vi "Verify.vi"(8 "error in (no error)":errorcluster, 10 "Comparator":refnum<class "Comparator.lvclass">, 11 "Mock In":refnum<class "Mock.lvclass">) -> (0 "error out":errorcluster, 1 "Errors":errorcluster[](array[cluster]), 2 "Results":cluster{"Passed?":bool, "Message":string}[](array[cluster]))   [LabVIEW 2020, in "Mock.lvclass"]
uses:
  Mock.lvclass
  Comparator/Comparator.lvclass
  Mock.lvclass/Mock.ctl
  Expectation/Expectation.lvclass
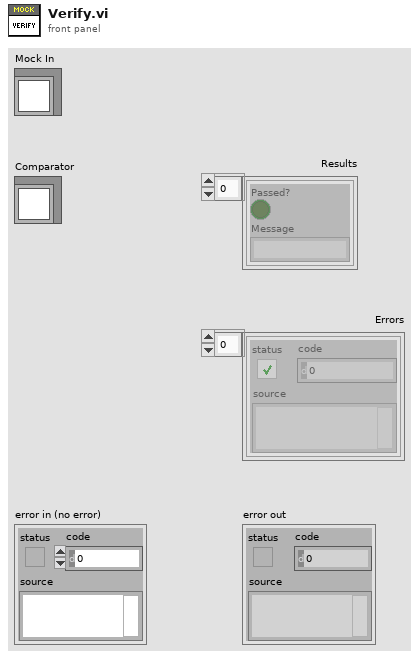
[diagram p1: front panel]
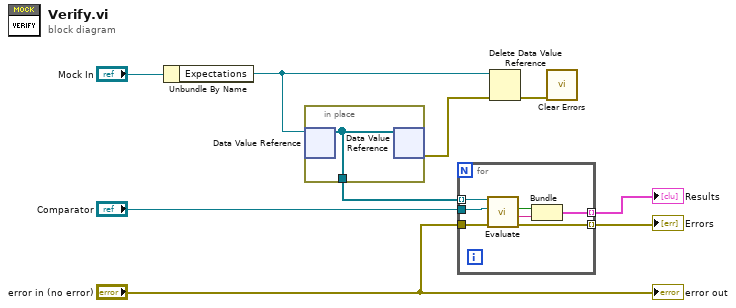
[diagram p0: block diagram]
diagram:
  n1 = Unbundle By Name("Mock In") -> ("Expectations"=w3:refnum<data-value>)
  n2 = in-place {
    in-place-border: [w10] -> w4
    n3 = in-place-dvr #1(w3) -> (w10:refnum<class "Expectation.lvclass">[])  [unwired: 1 out]
    n4 = in-place-dvr #1(w10) -> (w2:errorcluster)  [unwired: 1 out]
  }
  n5 = for {
    tunnel: "error in (no error)" -> [w17]
    tunnel: [w16] -> w7 mode=indexing
    tunnel: w4 -> [w15] mode=indexing
    tunnel: [w12] -> w6 mode=indexing
    tunnel: "Comparator" -> [w11]
    n6 = call-dynamic "Evaluate.vi"("error in (no error)"=w17, "Comparator"=w11, "Expectation in"=w15) -> ("error out"=w16:errorcluster, "Message"=w13:string, "Passed?"=w14:bool)  [unwired: 6 in]
    n7 = Bundle("Passed?"=w14, "Message"=w13) -> (w12:cluster{"Passed?":bool, "Message":string})  [unwired: 1 in]
  }
  "Errors" <- w7
  "Results" <- w6
  n8 = Delete Data Value Reference(data value reference=w3, error in=w2) -> (error out=w5:errorcluster)  [unwired: 1 out]
  n9 = call <vilib>:"Clear Errors.vi"("error in (no error)"=w5) -> ()  [unwired: 5 in, 2 out]
  "error out" <- "error in (no error)"
